vi "Read.vi"(11 "MessageQ Value in":refnum<class "MessageQ Value.lvclass">) -> (2 "MessageQ":refnum<class "MessageQ.lvclass">)   [LabVIEW 2020, in "Volatus.lvlib" / "MessageQ Value.lvclass"]
uses:
  MessageQ Value.lvclass
  MessageQ Value.lvclass/MessageQ Value.ctl
  MessageQ/MessageQ.lvclass
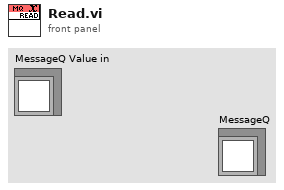
[diagram p1: front panel]
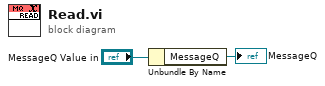
[diagram p0: block diagram]
diagram:
  n1 = Unbundle By Name("MessageQ Value in") -> ("MessageQ"=→"MessageQ":refnum<class "MessageQ.lvclass">)
